vi "freestream and source.vi"() -> ()   [LabVIEW 2025]
uses:
  <vilib>/Math Plots/3D Math Plots/3D Contour/3D Contour XCtrl/3D Contour.xctl
  <vilib>/Math Plots/3D Math Plots/3D Contour/3D Contour Datatype/Public/Plot Helper (Matrix).vi
  <vilib>/Math Plots/3D Math Plots/3D Contour/3D Contour Datatype/3D Contour Datatype.lvclass
panel:
  out "3D Contour":refnum<class "3D Plot Datatype.lvclass">[](xcontrol)
  in  "grid":i32
  in  "q_source":dbl
  in  "Source origin":cluster{"x":dbl, "y":dbl}
  in  "U infty":dbl
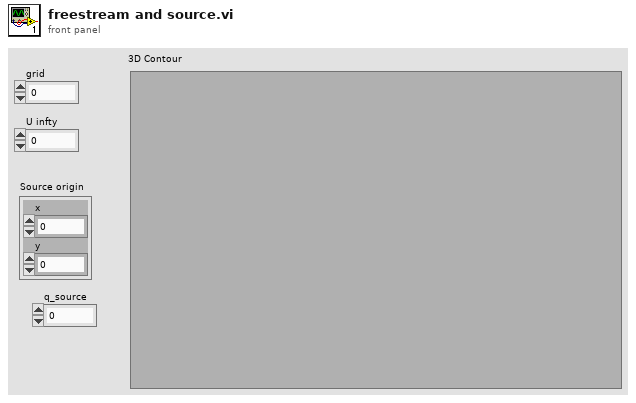
[diagram p1: front panel]
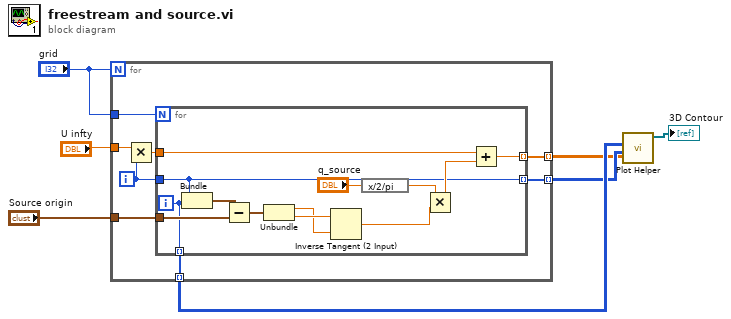
[diagram p0: block diagram]
diagram:
  n1 = for {
    N: "grid" -> [_]
    tunnel: "U infty" -> [w15]
    tunnel: "Source origin" -> [w13]
    tunnel: [w11] -> w1 mode=indexing
    tunnel: "grid" -> [w10]
    tunnel: [w9] -> w2 mode=indexing
    tunnel: [w8] -> w3 mode=indexing
    i -> [w14]
    n2 = Multiply(x=w15, y=w14) -> (x*y=w12:dbl)
    n3 = for {
      N: w10 -> [_]
      tunnel: w14 -> [w17]
      tunnel: w13 -> [w27]
      tunnel: w12 -> [w20]
      tunnel: [w18] -> w11 mode=indexing
      tunnel: [w17] -> w9 mode=indexing
      tunnel: [w16] -> w8 mode=indexing
      i -> [w16]
      n4 = Bundle(w17, w16) -> (w28:cluster{i32, i32})  [unwired: 1 in]
      n5 = Subtract(x=w28, y=w27) -> (x-y=w26:cluster{dbl, dbl})
      n6 = Unbundle(w26) -> (w24:dbl, w25:dbl)
      n7 = Inverse Tangent (2 Input)(1:w24, 2:w25) -> (0:w22:dbl)
      n8 = expression code="x/2/pi"("q_source") -> (w21:dbl)
      n9 = Multiply(x=w21, y=w22) -> (x*y=w19:dbl)
      n10 = Add(x=w20, y=w19) -> (x+y=w18:dbl)
    }
  }
  n11 = call-poly <vilib>:"Plot Helper.vi"("z matrix"=w1, "y matrix"=w2, "x matrix"=w3) -> ("3D Plot lvclass Array out"=→"3D Contour":refnum<class "3D Plot Datatype.lvclass">[])  [unwired: 3 in, 5 out]
